vi "refmgr_reset.vi"(8 "error in (no error)":errorcluster, 10 "RegExp":string, 11 "TagDB in":T1) -> (0 "error out":errorcluster, 1 "Keys":string[](array[string]), 3 "TagDB out":T1)   [LabVIEW 2014, in "RefManager(dev).lvlib"]
uses:
  RefManager(dev).lvlib
  <userlib>/_NEVSTOP/TagDB/Core/tagDB_Def.ctl
  <userlib>/_NEVSTOP/TagDB/Core/_Support/Error/_Clear Errors.vi
  <userlib>/_NEVSTOP/TagDB/Core/_Support/Properties/tagDB dbChanged.vi
  <userlib>/_NEVSTOP/TagDB/Core/_Support/Properties/tagDB getTags.vi
  <userlib>/_NEVSTOP/TagDB/Core/_Support/Access/_variant.vi
  <userlib>/_NEVSTOP/TagDB/Core/_XNode/tagDB_value.xnode/tagDB_value.xnode
  <userlib>/_NEVSTOP/TagDB/Core/TagDB.lvlib
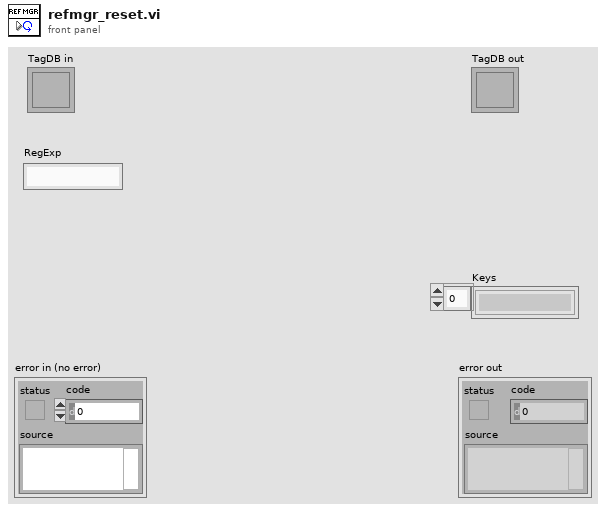
[diagram p1: front panel]
types:
  T1 = typedef "TagDB.lvlib/tagDB_Def.ctl" = refnum<k1>
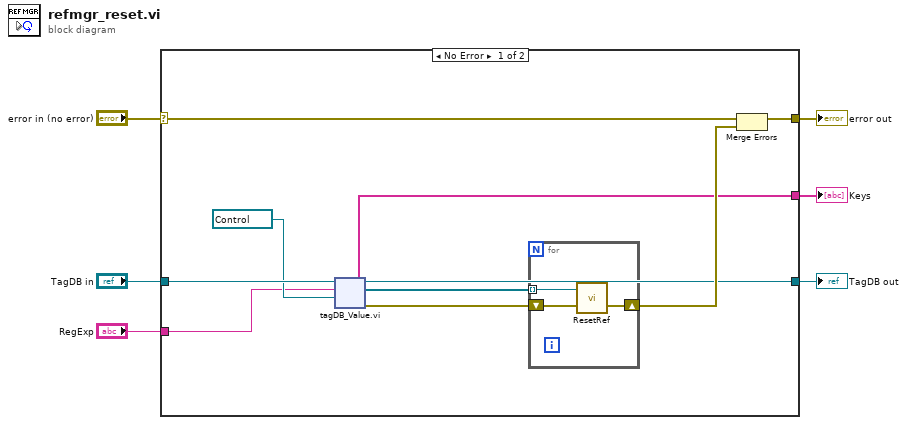
[diagram p0: block diagram]
diagram:
  n1 = case shown="No Error" "error in (no error)" {
    selector: "error in (no error)" -> [w15 w120]
    tunnel: [w16 w120] -> w6
    tunnel: "TagDB in" -> [w13 w119]
    tunnel: "RegExp" -> [w11 _]
    tunnel: [w7 _] -> w2
    tunnel: [w8 w119] -> w1
    frame No Error {
      n2 = xnode "tagDB_Value.vi"("DB Ref"=w13, "Type"=refnum<vi> refnum, "RegExp"=w11) -> ("error out"=w9:errorcluster, "DB Ref(dup)"=w8:T1, "value"=w10:refnum<vi>[], "names"=w7:string[])  [unwired: 1 in]
      n3 = for {
        tunnel: w10 -> [w118] mode=indexing
        shift-right: [w116] -> w14
        shift-left: w9 -> [w117]
        n4 = call "ResetRef.vi"("error in (no error)"=w117, "Boolean in"=w118) -> ("error out"=w116:errorcluster)  [unwired: 8 in, 1 out]
      }
      n5 = Merge Errors(w15, w14) -> (w16:errorcluster)
    }
    frame Error {
    }
  }
  "error out" <- w6
  "TagDB out" <- w1
  "Keys" <- w2
